vi "set_position.vi"(8 "error in (no error)":errorcluster, 10 "last position":dbl, 11 "imaginaryStage in":refnum<class "imaginaryStage.lvclass">) -> (0 "error out":errorcluster, 3 "imaginaryStage out":refnum<class "imaginaryStage.lvclass">)   [LabVIEW 2018, in "imaginaryStage.lvclass"]
uses:
  imaginaryStage.lvclass
  _delayStageBase/_delayStageBase.lvclass
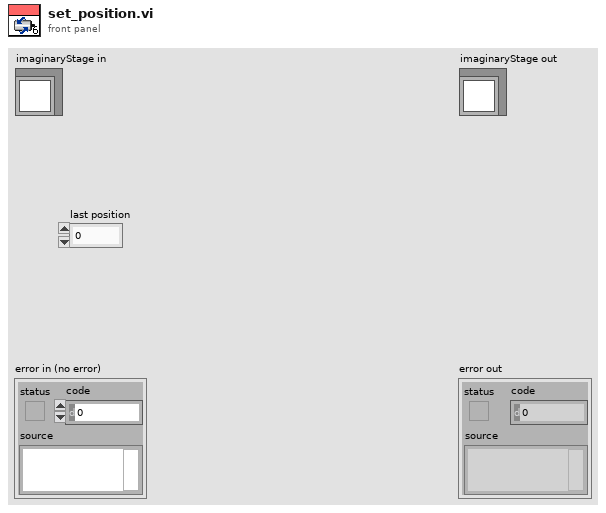
[diagram p1: front panel]
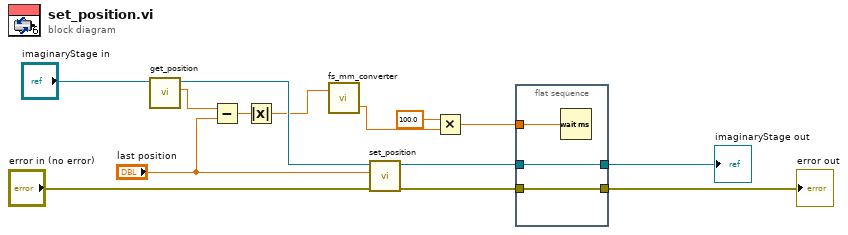
[diagram p0: block diagram]
diagram:
  n1 = call-dynamic "get_position.vi"("_delayStageBase in"="imaginaryStage in") -> ("last position"=w11:dbl, "_delayStageBase out"=w12:refnum<class "imaginaryStage.lvclass">)  [unwired: 8 in, 1 out]
  n2 = Subtract(x=w11, y="last position") -> (x-y=w9:dbl)
  n3 = Absolute Value(x=w9) -> (abs(x)=w2:dbl)
  n4 = call "fs_mm_converter.vi"("fs in"=w2) -> ("mm out"=w1:dbl)  [unwired: 1 in, 1 out]
  n5 = call-parent "set_position.vi"("error in (no error)"="error in (no error)", "last position"="last position", "_delayStageBase in"=w12) -> ("error out"=w5:errorcluster, "_delayStageBase out"=w8:refnum<class "imaginaryStage.lvclass">)  [unwired: 7 in]
  n6 = Multiply(x=100.0, y=w1) -> (x*y=w4:dbl)
  n7 = flat-sequence {
    tunnel: w8 -> [w17]
    tunnel: [w17] -> w7
    tunnel: [w16] -> w6
    tunnel: w5 -> [w16]
    tunnel: w4 -> [w15]
    frame #0 {
      n8 = Wait (ms)(milliseconds to wait=w15) -> ()  [unwired: 1 out]
    }
  }
  "error out" <- w6
  "imaginaryStage out" <- w7
